vi "servoOpen (SubVI).vi"() -> (0 "error out":errorcluster, 3 "ServosRef":refnum<class "PWM Generator.lvclass">[](array[class]))   [LabVIEW 2020]
uses:
  <vilib>/CISH Robotics/L4VMX VMXpi/PWM Generator/PWM Generator.lvclass
  <vilib>/CISH Robotics/L4VMX VMXpi/Type Def/VMX Channel Index.ctl
  <vilib>/CISH Robotics/L4VMX VMXpi/L4VMX.lvlib
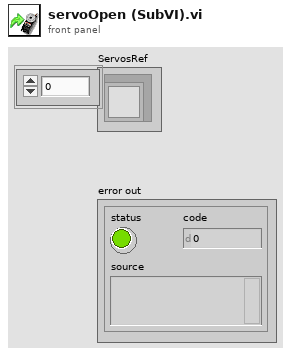
[diagram p1: front panel]
types:
  T1 = typedef "L4VMX.lvlib/VMX Channel Index.ctl" = enum16{"0", "1", "2", "3", "4", "5", "6", "7", "8", "9", "10", "11", "12", "13", "14", "15", "16", "17", "18", "19", "20", "21", "22", "23", "24", "25", "26", "27", "28", "29", "30", "31", "32", "33"}
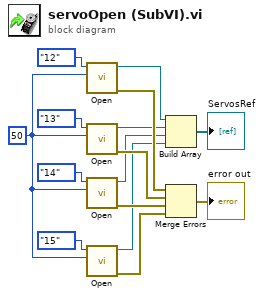
[diagram p0: block diagram]
diagram:
  w5 = u32 50 ("Frequency(Hz)")
  n1 = call <vilib>:"Open.vi"("Frequency(Hz)"=w5, "VMX Channel Index"=VMX_Channel_Index."12") -> ("Error Out"=w11:errorcluster, "PWM Generator Object"=w6:refnum<class "PWM Generator.lvclass">)  [unwired: 8 in]
  n2 = call <vilib>:"Open.vi"("Frequency(Hz)"=w5, "VMX Channel Index"=VMX_Channel_Index."13") -> ("Error Out"=w12:errorcluster, "PWM Generator Object"=w7:refnum<class "PWM Generator.lvclass">)  [unwired: 8 in]
  n3 = call <vilib>:"Open.vi"("Frequency(Hz)"=w5, "VMX Channel Index"=VMX_Channel_Index."14") -> ("Error Out"=w13:errorcluster, "PWM Generator Object"=w8:refnum<class "PWM Generator.lvclass">)  [unwired: 8 in]
  n4 = call <vilib>:"Open.vi"("Frequency(Hz)"=w5, "VMX Channel Index"=VMX_Channel_Index."15") -> ("Error Out"=w14:errorcluster, "PWM Generator Object"=w9:refnum<class "PWM Generator.lvclass">)  [unwired: 8 in]
  n5 = Build Array(w6, w7, w8, w9) -> (→"ServosRef":refnum<class "PWM Generator.lvclass">[])
  n6 = Merge Errors(w11, w12, w13, w14) -> (→"error out":errorcluster)
